vi "WLAN_TDMA_FrameBuild.vi"(8 "error in (no error)":errorcluster, 9 "data in 2":i8[](array[numeric]) caption="input bit stream", 10 "Modulation parameter":T1, 11 "data in":i8[](array[numeric]) caption="input bit stream") -> (0 "error out":errorcluster, 2 "output symbols":cdb[](array[numeric]), 3 "output array":cdb[](array[numeric]))   [LabVIEW 2022 SP3]
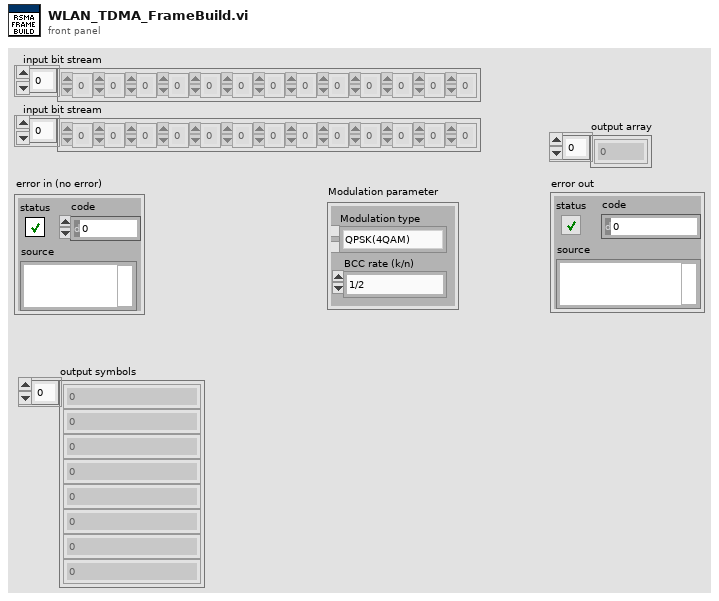
[diagram p1: front panel]
types:
  T1 = cluster{"Modulation type":enum16{"QPSK(4QAM)", "64QAM", "16QAM", "BPSK"}, "BCC rate (k/n)":enum16{"1/2", "2/3", "3/4"}}
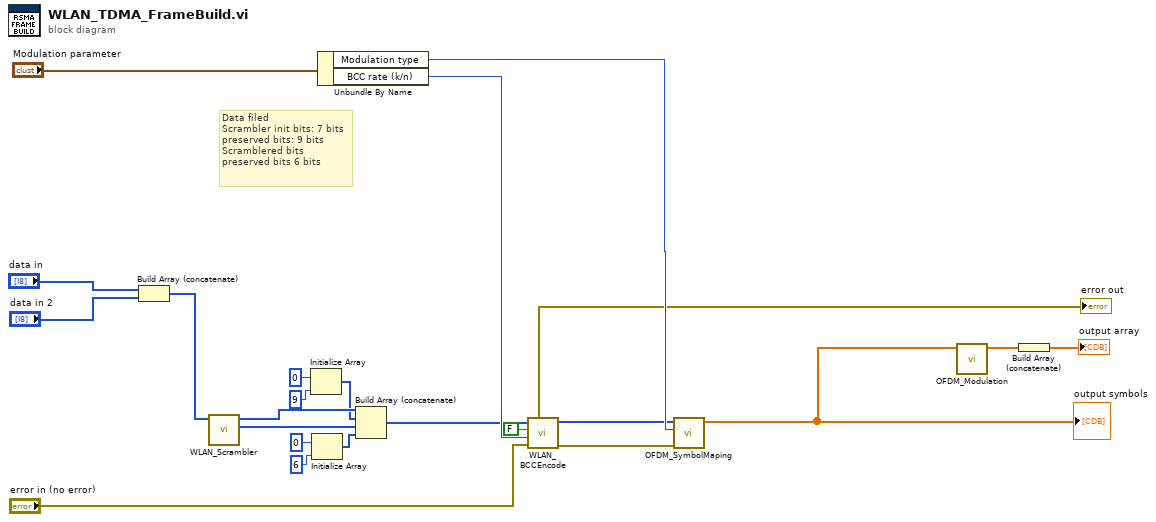
[diagram p0: block diagram]
diagram:
  # "Data filed\nScrambler init bits: 7 bits\npreserved bits: 9 bits\nScramblered bits\npreserved bits 6 bits"
  n1 = Build Array (concatenate)("data in", "data in 2") -> (w5:i8[])
  n2 = call "WLAN_Scrambler.vi"("input bit stream"=w5) -> ("scrambled bits"=w11:i8[], "scrambler initial bit"=w15:i8[])  [unwired: 9 in]
  n3 = Initialize Array(i8 0 ("element"), 9 ("dimension size")) -> (w14:i8[])
  n4 = Initialize Array(i8 0 ("element"), 6 ("dimension size")) -> (w8:i8[])
  n5 = Unbundle By Name("Modulation parameter") -> ("Modulation type"=w21:enum16{"QPSK(4QAM)", "64QAM", "16QAM", "BPSK"}, "BCC rate (k/n)"=w20:enum16{"1/2", "2/3", "3/4"})
  n6 = Build Array (concatenate)(w15, w14, w11, w8) -> (w18:i8[])
  n7 = call "WLAN_BCCEncode.vi"("error in (no error)"="error in (no error)", "BCC rate (k/n)"=w20, "need add zeros?"=FALSE, "input bit stream"=w18) -> ("error out"=w16:errorcluster, "output bit stream 3"=w17:i8[])  [unwired: 6 in]
  n8 = call "OFDM_SymbolMaping.vi"("error in (no error)"=w16, "Modulation type"=w21, "input bit stream"=w17) -> ("symbols"=w1:cdb[])  [unwired: 7 in, 1 out]
  "output symbols" <- w1
  n9 = call "OFDM_Modulation.vi"("Input sequence"=w1) -> ("Output sequence"=w6:cdb[])  [unwired: 10 in]
  n10 = Build Array (concatenate)(w6) -> (→"output array":cdb[])
  "error out" <- "error in (no error)"
